vi "Actor Core.vi"(8 "error in":errorcluster caption="错误输入", 11 "MiddleMasterActor in":refnum<class "MiddleMasterActor.lvclass"> caption="操作者输入") -> (0 "error out":errorcluster caption="错误输出", 3 "Actor out":refnum<class "Actor.lvclass"> caption="操作者输出")   [LabVIEW 2014, in "UnitTest.lvlib" / "MiddleMasterActor.lvclass"]
doc: "(<B>文件名</B>：Actor Framework.lvlib:Actor.lvclass:Actor Core.vi)\n\n接收发送至操作者的消息，响应消息并处理可能导致操作者关闭的错误。\n\n子孙类重写该VI，使操作者完成特定的任务。使用调用父方法节点实现重写。"
uses:
  MiddleMasterActor.lvclass
  <vilib>/ActorFramework/Actor/Actor.lvclass
  <vilib>/ActorFramework/Actor/Actor.lvclass/Actor.ctl
  <vilib>/ActorFramework/Message Enqueuer/Message Enqueuer.lvclass/Message Enqueuer.ctl
  <vilib>/ActorFramework/Message Enqueuer/Enqueue.vi
  <vilib>/ActorFramework/Message Priority Queue/Priority Enqueue.vi
  <vilib>/ActorFramework/Stop Msg/Stop Msg.lvclass
panel:
  in  "停止按钮":bool
  in  "SlaveStart":bool
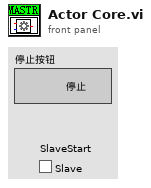
[diagram p1: front panel]
types:
  T1 = enum16{"OpenSlaveActor", "Idle", "StopSlaveActor"}
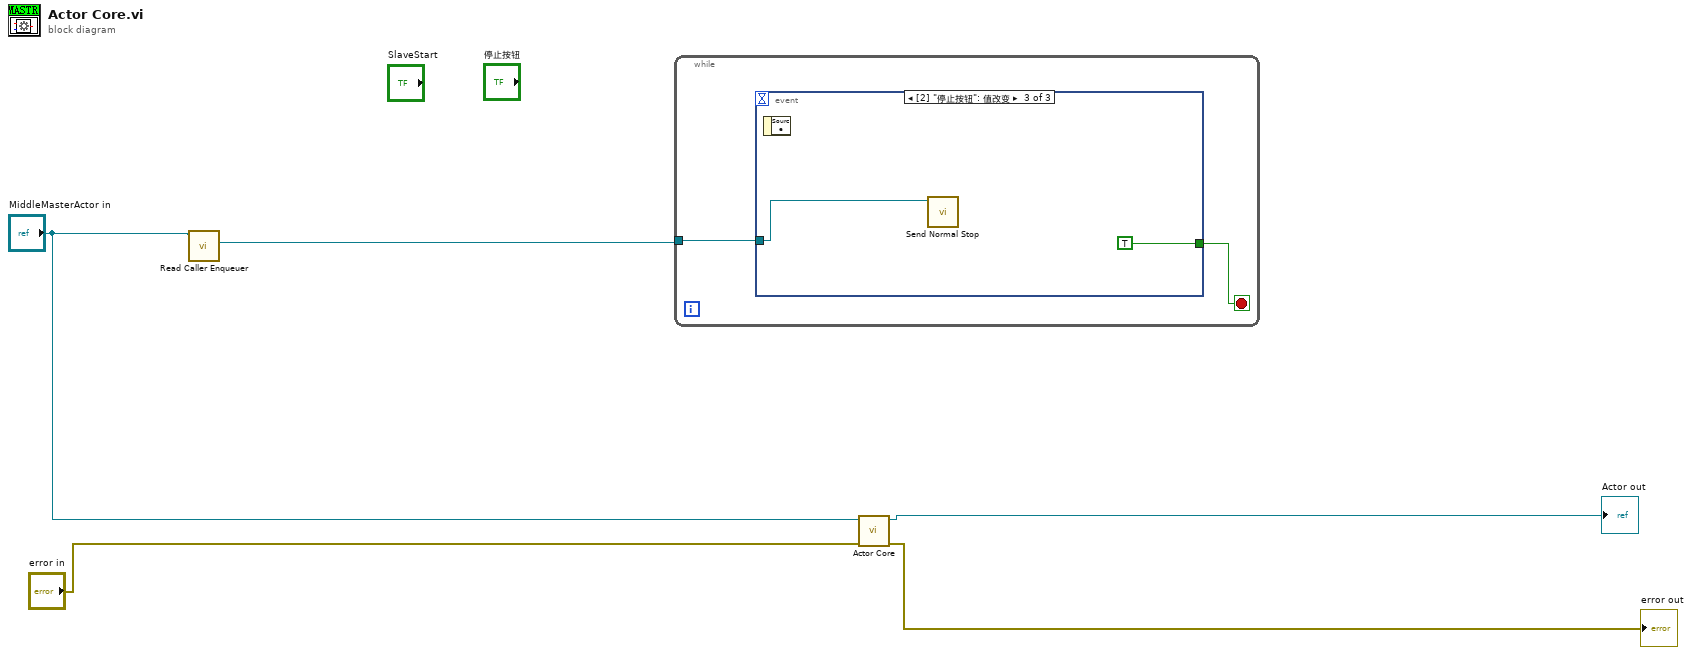
[diagram p0: block diagram]
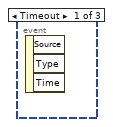
[diagram p2: hidden frame]
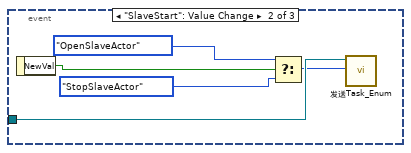
[diagram p3: hidden frame]
diagram:
  n1 = call <vilib>:"Read Caller Enqueuer.vi"("Actor"="MiddleMasterActor in") -> ("Caller Enqueuer"=w1:refnum<class "Message Enqueuer.lvclass">)  [unwired: 10 in]
  n2 = while {
    tunnel: w1 -> [w7]
    stop <- w6 stop-if-true
    n3 = event shown="[2] \"停止按钮\": 值改变" {
      selector: _ -> [_ _ _]
      dyn-events: _ -> [_ _ _]
      timeout: _ -> [_ _ _]
      tunnel: w7 -> [_ w12 w14]
      tunnel: [_ _ TRUE] -> w6
      event Timeout {
        n4 = event-data() -> ()  [unwired: 1 in, 3 out]
      }
      event "SlaveStart": Value Change {
        n5 = event-data() -> ("NewVal"=w11:bool)  [unwired: 1 in]
        n6 = Select(t=T1."OpenSlaveActor" ("Enum"), s=w11, f=T1."StopSlaveActor" ("Enum")) -> (s? t:f=w10:T1)
        n7 = call "发送Task_Enum.vi"("Enum"=w10, "消息待入队列"=w12) -> ()  [unwired: 8 in, 2 out]
      }
      event "停止按钮": Value Change {
        n8 = event-data() -> ()  [unwired: 1 in, 1 out]
        n9 = call <vilib>:"Send Normal Stop.vi"("Message Enqueuer"=w14) -> ()  [unwired: 10 in, 1 out]
      }
    }
  }
  n10 = call-parent "Actor Core.vi"("error in"="error in", "Actor in"="MiddleMasterActor in") -> ("error out"=→"error out":errorcluster, "Actor out"=→"Actor out":refnum<class "Actor.lvclass">)  [unwired: 8 in]
